vi "Teleop.vi"(0 "Call Context":T10) -> (6 "SubState 3":T4, 8 "SubState 4":T4, 9 "SubState 5":T9, 11 "Loop 3 Data":T5, 13 "Loop 4 Data":T3, 14 "SubState 0":T4=enum."driver control", 15 "Loop 1 Data":T7, 16 "Loop 0 Data":T8, 17 "SubState 1":T4, 18 "Loop 2 Data":T6, 19 "SubState 2":T4)   [LabVIEW 2013]
uses:
  typedefs/subStates.ctl
  <vilib>/Rock Robotics/WPI/DriverStation/WPI_DriverStationDerivedRobotMode.ctl
  typedefs/singleUseSubstate.ctl
  typedefs/Loop Datatypes/Loop 0 Datatype.ctl
  typedefs/Loop Datatypes/Loop 1 Datatype.ctl
  typedefs/Loop Datatypes/Loop 2 Datatype.ctl
  typedefs/Loop Datatypes/Loop 3 Datatype.ctl
  typedefs/Loop Datatypes/Loop 4 Datatype.ctl
  <vilib>/Rock Robotics/WPI/Joystick/WPI_JoystickDevRef.ctl
  <vilib>/Rock Robotics/WPI/Joystick/WPI_JoystickDeviceEnum.ctl
  typedefs/fg_typedef.ctl
  <vilib>/Rock Robotics/WPI/Joystick/WPI_JoystickGetSetRefNum.vi
panel:
  out "Drive to DC":bool
  out "JS2 Button 9":bool
  out "JS3":T1
  out "JS1":T1
  out "JS2":T1
  out "Exit Value":i32=-1
  # "Loop Data and Substates"
  # "Drive Loop"
  # "Unassigned Loop"
  # "Unassigned Loop"
  # "Unassigned Loop"
  # "Unassigned Loop"
  # "Pneumatic Loop"
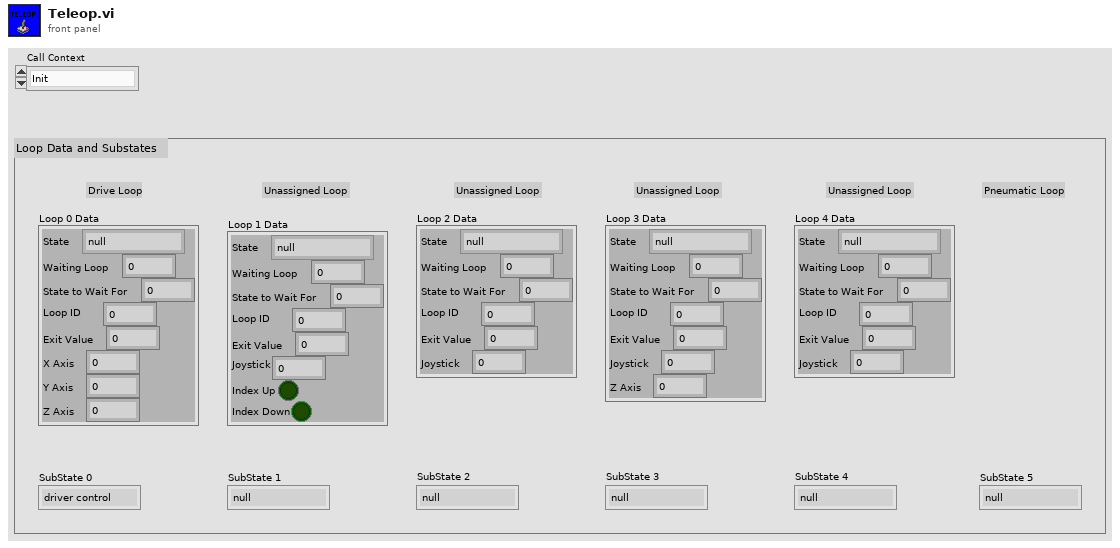
[diagram p1: front panel]
types:
  T1 = typedef "WPI_JoystickDevRef.ctl" = cluster{"Device":T2}
  T2 = typedef "WPI_JoystickDeviceEnum.ctl" = enum16{"USB 1", "USB 2", "USB 3", "USB 4", "Kinect 1", "Kinect 2"}
  T3 = typedef "Loop 4 Datatype.ctl" = cluster{"State":T4, "Waiting Loop":i32, "State to Wait For":i32, "Loop ID":i32, "Exit Value":i32, "Joystick":dbl}
  T4 = typedef "subStates.ctl" = enum16{"null", "wait", "driver control", "auto", "manual override", "hold position", "rotate", "feeder", "shoot", "end"}
  T5 = typedef "Loop 3 Datatype.ctl" = cluster{"State":T4, "Waiting Loop":i32, "State to Wait For":i32, "Loop ID":i32, "Exit Value":i32, "Joystick":dbl, "Z Axis":dbl}
  T6 = typedef "Loop 2 Datatype.ctl" = cluster{"State":T4, "Waiting Loop":i32, "State to Wait For":i32, "Loop ID":i32, "Exit Value":i32, "Joystick":dbl}
  T7 = typedef "Loop 1 Datatype.ctl" = cluster{"State":T4, "Waiting Loop":i32, "State to Wait For":i32, "Loop ID":i32, "Exit Value":i32, "Joystick":dbl, "Index Up":bool, "Index Down":bool}
  T8 = typedef "Loop 0 Datatype.ctl" = cluster{"State":T4, "Waiting Loop":i32, "State to Wait For":i32, "Loop ID":i32, "Exit Value":i32, "X Axis":dbl, "Y Axis":dbl, "Z Axis":dbl}
  T9 = typedef "singleUseSubstate.ctl" = enum16{"null", "wait", "shift high", "shift low"}
  T10 = typedef "WPI_DriverStationDerivedRobotMode.ctl" = enum16{"Init", "Execute", "Stop"}
  T11 = cluster{"axis 1 (x)":dbl, "axis 2 (y)":dbl, "axis 3 (throttle)":dbl, "axis 4":dbl, "axis 5":dbl, "axis 6":dbl}
  T12 = typedef "WPI_JoystickButtonState.ctl" = cluster{"Button 1":bool, "Button 2":bool, "Button 3":bool, "Button 4":bool, "Button 5":bool, "Button 6":bool, "Button 7":bool, "Button 8":bool, "Button 9":bool, "Button 10":bool, "Button 11":bool, "Button 12":bool}
  T13 = typedef "WPI_EncoderDevRef.ctl" = cluster{"DevStatus":errorcluster, "EncoderIndex":T14, "CounterIndex":T15, "DistancePerCount":dbl, "Decoding Type":T16}
  T14 = typedef "FPGA_EncoderIdx.ctl" = enum8{"Enc 0", "Enc 1", "Enc 2", "Enc 3", "Invalid"}
  T15 = typedef "FPGA_CounterCtrSystemIndex.ctl" = enum8{"Ctr 0", "Ctr 1", "Ctr 2", "Ctr 3", "Ctr 4", "Ctr 5", "Ctr 6", "Ctr 7", "Invalid"}
  T16 = typedef "WPI_EncoderType.ctl" = enum16{"1x", "2x", "4x"}
  T17 = typedef "fg_typedef.ctl" = enum16{"Get", "Set"}
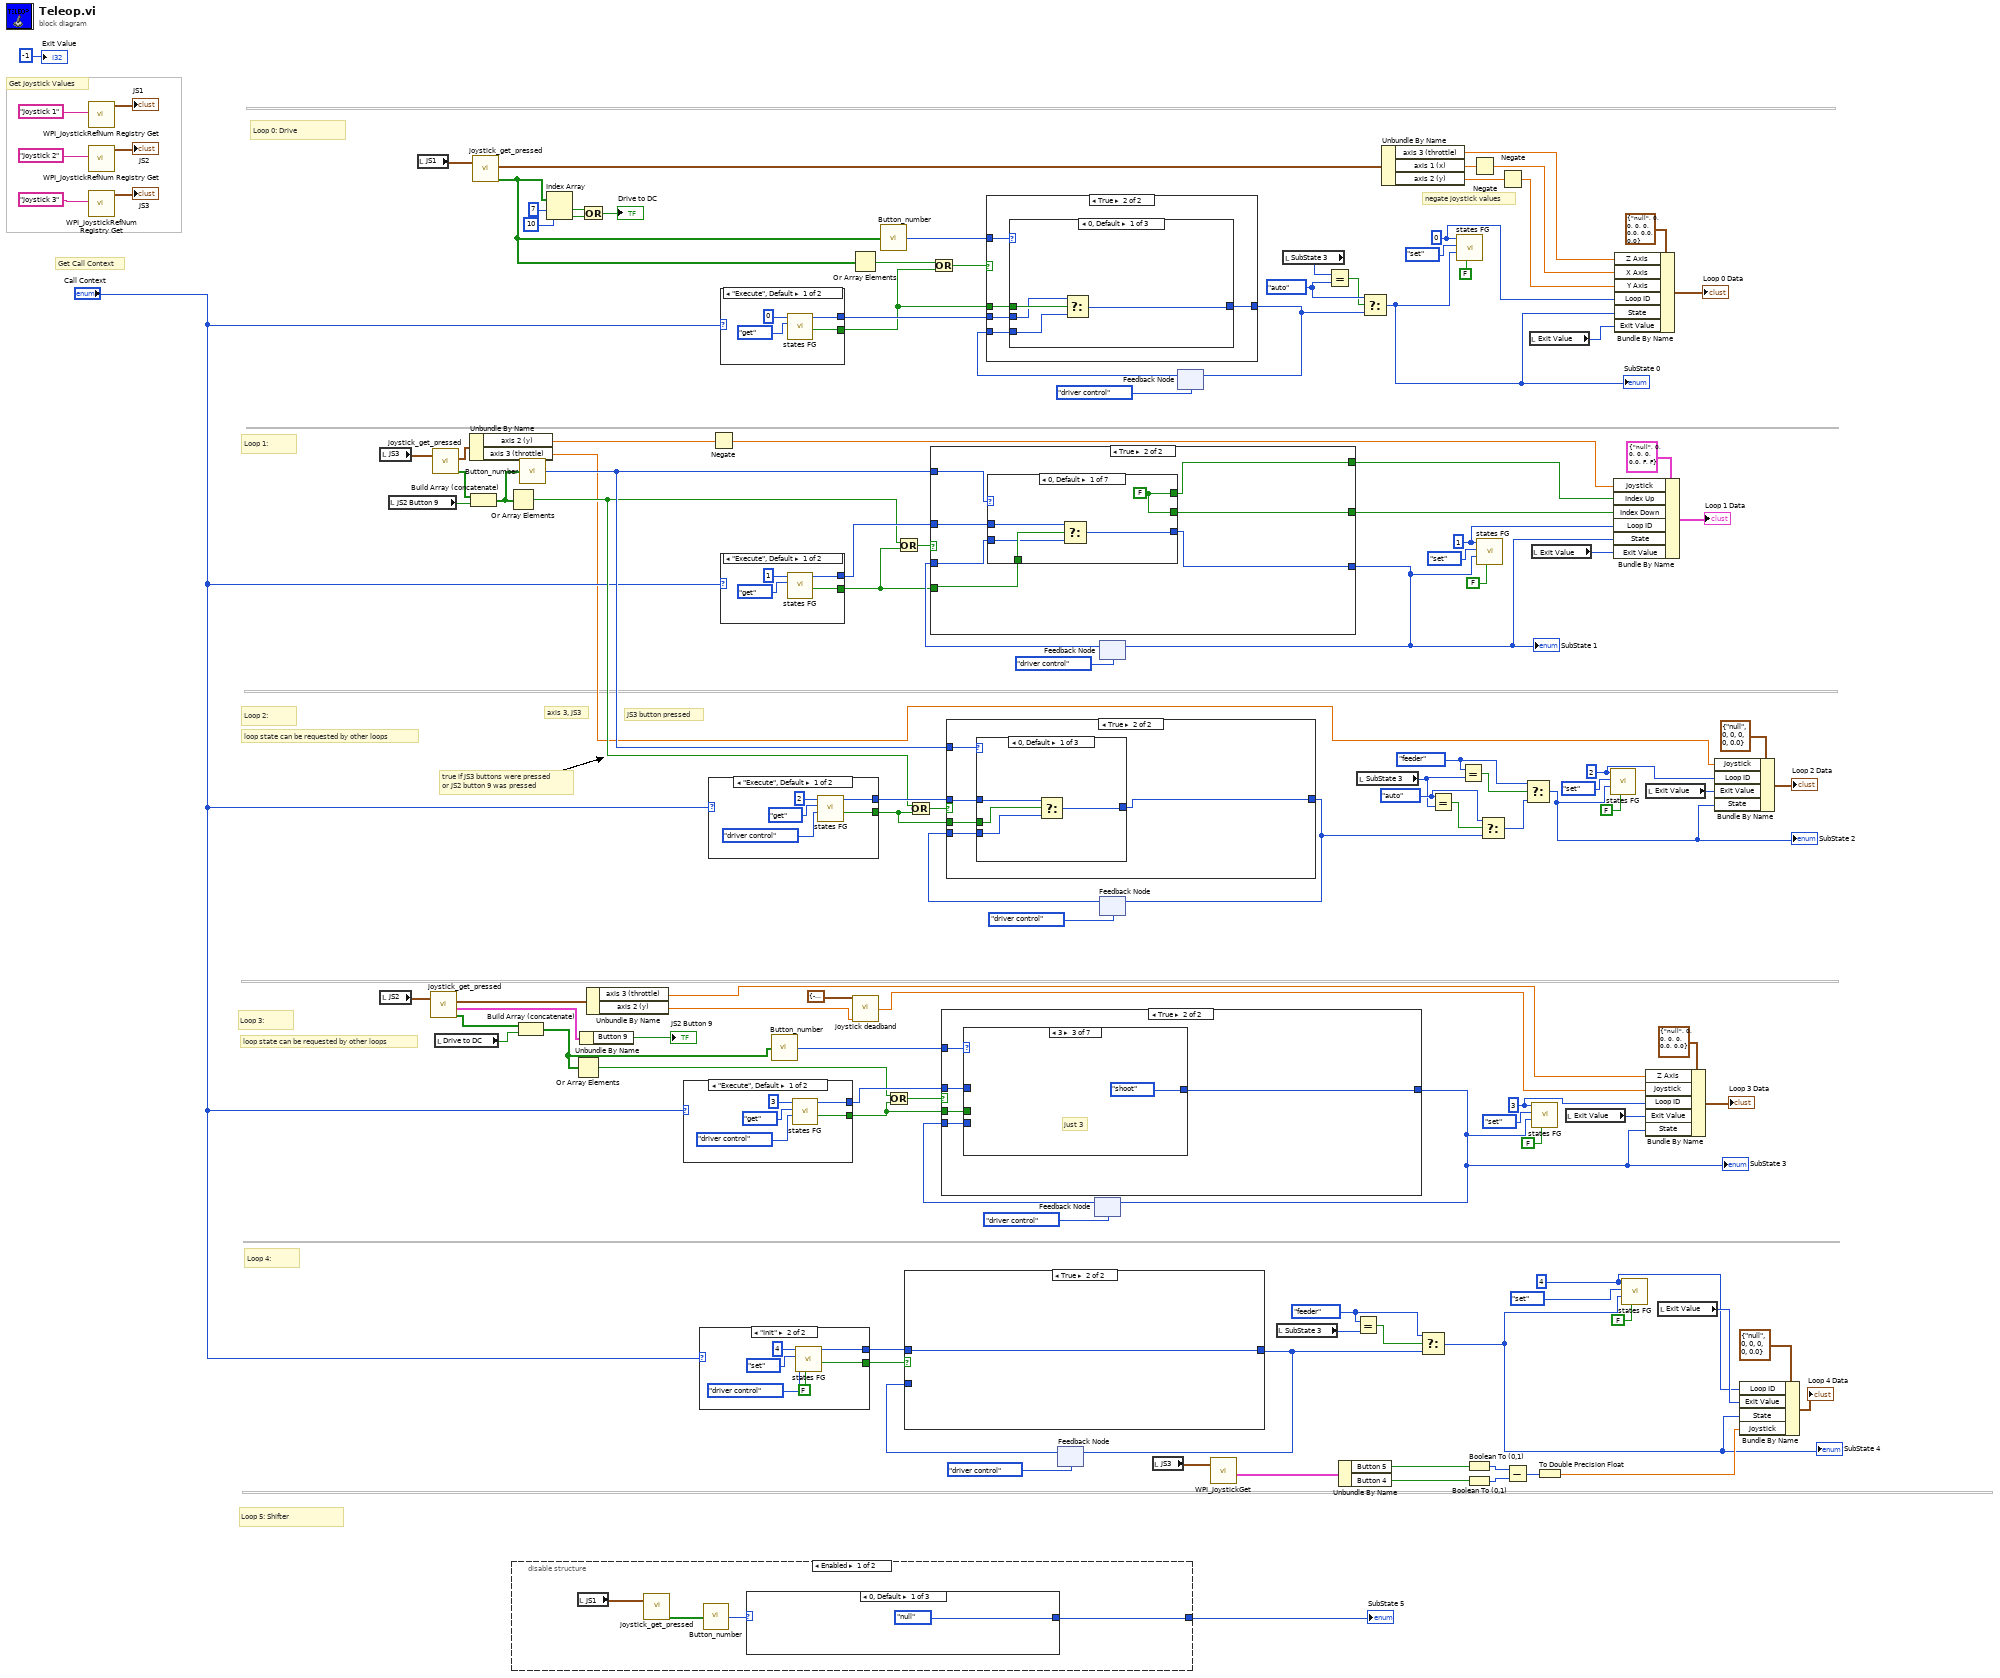
[diagram p0: block diagram]
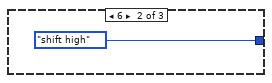
[diagram p2: hidden frame]
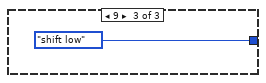
[diagram p3: hidden frame]
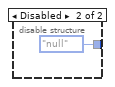
[diagram p4: hidden frame]
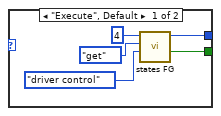
[diagram p6: hidden frame]
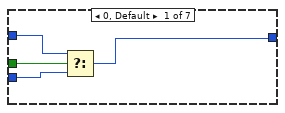
[diagram p8: hidden frame]
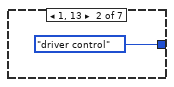
[diagram p9: hidden frame]
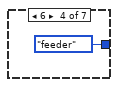
[diagram p10: hidden frame]
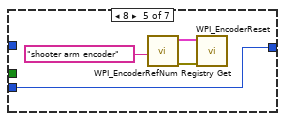
[diagram p11: hidden frame]
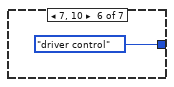
[diagram p12: hidden frame]
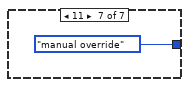
[diagram p13: hidden frame]
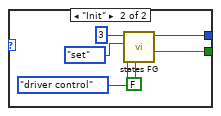
[diagram p14: hidden frame]
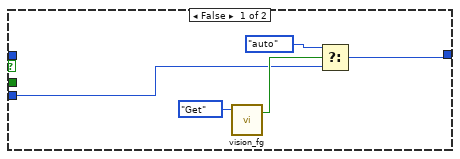
[diagram p15: hidden frame]
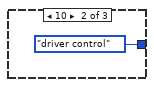
[diagram p16: hidden frame]
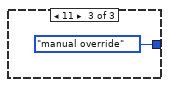
[diagram p17: hidden frame]
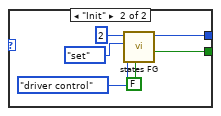
[diagram p18: hidden frame]
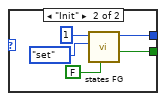
[diagram p19: hidden frame]
diagram:
  w23 = subStates."auto" ("y")
  w26 = subStates."auto" ("x")
  w33 = subStates."feeder" ("x")
  w35 = subStates."feeder" ("x")
  w88 = 4 ("Loop ID")
  w103 = 3 ("Loop ID")
  w104 = 2 ("Loop ID")
  w113 = 1 ("Loop ID")
  w115 = 0 ("Loop ID")
  # "true if JS3 buttons were pressed\nor JS2 button 9 was pressed"
  # "JS3 button pressed"
  # "axis 3, JS3"
  # "negate joystick values"
  # "Get Call Context"
  # "Get Joystick Values"
  # "Loop 4:"
  # "Loop 3:"
  # "loop state can be requested by other loops"
  # "Loop 5: Shifter"
  # "Loop 2:"
  # "Loop 1:"
  # "Loop 0: Drive"
  # "loop state can be requested by other loops"
  n1 = call <vilib>:"WPI_JoystickRefNum Registry Get.vi"("refnum name"="Joystick 1") -> ("JoystickDevRef"=→"JS1":T1)  [unwired: 9 in, 1 out]
  n2 = call <vilib>:"WPI_JoystickRefNum Registry Get.vi"("refnum name"="Joystick 2") -> ("JoystickDevRef"=→"JS2":T1)  [unwired: 9 in, 1 out]
  n3 = call <vilib>:"WPI_JoystickRefNum Registry Get.vi"("refnum name"="Joystick 3") -> ("JoystickDevRef"=→"JS3":T1)  [unwired: 9 in, 1 out]
  n4 = local read "JS3"() -> (w68:T1)
  n5 = local read "JS2"() -> (w46:T1)
  n6 = local read "JS2 Button 9"() -> (w53:bool)
  n7 = local read "JS1"() -> (w69:T1)
  n8 = call "joystick_get_pressed.vi"("JoystickDevRef 2"=w46) -> ("Axes"=w51:T11, "Buttons"=w5:T12, "Buttons Pressed?"=w49:bool[])  [unwired: 1 in, 1 out]
  n9 = call "joystick_get_pressed.vi"("JoystickDevRef 2"=w68) -> ("Axes"=w67:T11, "Buttons Pressed?"=w29:bool[])  [unwired: 1 in, 2 out]
  n10 = local read "Drive to DC"() -> (w8:bool)
  n11 = Unbundle By Name(w67) -> ("axis 2 (y)"=w76:dbl, "axis 3 (throttle)"=w3:dbl)
  n12 = Build Array (concatenate)(w29, w53) -> (w28:bool[])
  n13 = call "joystick_get_pressed.vi"("JoystickDevRef 2"=w69) -> ("Axes"=w75:T11, "Buttons Pressed?"=w14:bool[])  [unwired: 1 in, 2 out]
  n14 = Or Array Elements(Boolean array=w28) -> (logical OR=w56:bool)
  n15 = disable-structure shown="Enabled" {
    disable-tunnel: [w133 singleUseSubstate."null" ("SubState 5")] -> w85
    frame Enabled {
      n16 = local read "JS1"() -> (w132:T1)
      n17 = call "joystick_get_pressed.vi"("JoystickDevRef 2"=w132) -> ("Buttons Pressed?"=w135:bool[])  [unwired: 1 in, 3 out]
      n18 = call "Button_number.vi"("Button Array"=w135) -> ("Button Pressed"=w134:i32)
      n19 = case shown="0, Default" w134 {
        tunnel: [singleUseSubstate."null" ("Enum") singleUseSubstate."shift high" ("Enum") singleUseSubstate."shift low" ("Enum")] -> w133
        frame 0, Default {
        }
        frame 6 {
        }
        frame 9 {
        }
      }
    }
    frame Disabled {
    }
  }
  "SubState 5" <- w85
  n20 = Build Array (concatenate)(w49, w8) -> (w2:bool[])
  n21 = call "Button_number.vi"("Button Array"=w28) -> ("Button Pressed"=w58:i32)
  n22 = Index Array(array=w14, index #1=7 ("index"), index #2=10 ("index")) -> (element #1=w11:bool, element #2=w10:bool)
  n23 = Or Array Elements(Boolean array=w2) -> (logical OR=w50:bool)
  n24 = Unbundle By Name(w5) -> ("Button 9"=→"JS2 Button 9":bool)
  n25 = Or(x=w11, y=w10) -> (x .or. y?=→"Drive to DC":bool)
  n26 = Unbundle By Name(w51) -> ("axis 3 (throttle)"=w16:dbl, "axis 2 (y)"=w19:dbl)
  n27 = case shown="\"Execute\", Default" "Call Context" {
    tunnel: [w142 w148] -> w47
    tunnel: [w140 w145] -> w101
    frame "Execute", Default {
      n28 = call "states FG.vi"("subState in"=subStates."driver control", "menu (get)"=enum16{"set", "get"}."get", "Loop ID"=3) -> ("exit out"=w142:bool, "subState out"=w140:T4)  [unwired: 5 in, 2 out]
    }
    frame "Init" {
      n29 = call "states FG.vi"("exit in"=FALSE, "subState in"=subStates."driver control", "menu (get)"=enum16{"set", "get"}."set", "Loop ID"=3) -> ("exit out"=w148:bool, "subState out"=w145:T4)  [unwired: 4 in, 2 out]
    }
  }
  n30 = case shown="\"Init\"" "Call Context" {
    tunnel: [w153 w159] -> w43
    tunnel: [w151 w156] -> w90
    frame "Execute", Default {
      n31 = call "states FG.vi"("subState in"=subStates."driver control", "menu (get)"=enum16{"set", "get"}."get", "Loop ID"=4) -> ("exit out"=w153:bool, "subState out"=w151:T4)  [unwired: 5 in, 2 out]
    }
    frame "Init" {
      n32 = call "states FG.vi"("exit in"=FALSE, "subState in"=subStates."driver control", "menu (get)"=enum16{"set", "get"}."set", "Loop ID"=4) -> ("exit out"=w159:bool, "subState out"=w156:T4)  [unwired: 4 in, 2 out]
    }
  }
  n33 = case shown="\"Execute\", Default" "Call Context" {
    tunnel: [w164 w170] -> w55
    tunnel: [w162 w167] -> w120
    frame "Execute", Default {
      n34 = call "states FG.vi"("subState in"=subStates."driver control", "menu (get)"=enum16{"set", "get"}."get", "Loop ID"=2) -> ("exit out"=w164:bool, "subState out"=w162:T4)  [unwired: 5 in, 2 out]
    }
    frame "Init" {
      n35 = call "states FG.vi"("exit in"=FALSE, "subState in"=subStates."driver control", "menu (get)"=enum16{"set", "get"}."set", "Loop ID"=2) -> ("exit out"=w170:bool, "subState out"=w167:T4)  [unwired: 4 in, 2 out]
    }
  }
  n36 = Negate(x=w76) -> (-x=w61:dbl)
  n37 = case shown="\"Execute\", Default" "Call Context" {
    tunnel: [w174 w179] -> w65
    tunnel: [w173 w177] -> w118
    frame "Execute", Default {
      n38 = call "states FG.vi"("menu (get)"=enum16{"set", "get"}."get", "Loop ID"=0) -> ("exit out"=w174:bool, "subState out"=w173:T4)  [unwired: 6 in, 2 out]
    }
    frame "Init" {
      n39 = call "states FG.vi"("exit in"=FALSE, "menu (get)"=enum16{"set", "get"}."set", "Loop ID"=0) -> ("exit out"=w179:bool, "subState out"=w177:T4)  [unwired: 5 in, 2 out]
    }
  }
  n40 = case shown="\"Execute\", Default" "Call Context" {
    tunnel: [w183 w188] -> w62
    tunnel: [w182 w186] -> w117
    frame "Execute", Default {
      n41 = call "states FG.vi"("menu (get)"=enum16{"set", "get"}."get", "Loop ID"=1) -> ("exit out"=w183:bool, "subState out"=w182:T4)  [unwired: 6 in, 2 out]
    }
    frame "Init" {
      n42 = call "states FG.vi"("exit in"=FALSE, "menu (get)"=enum16{"set", "get"}."set", "Loop ID"=1) -> ("exit out"=w188:bool, "subState out"=w186:T4)  [unwired: 5 in, 2 out]
    }
  }
  n43 = call "Button_number.vi"("Button Array"=w2) -> ("Button Pressed"=w48:i32)
  n44 = Or Array Elements(Boolean array=w14) -> (logical OR=w66:bool)
  n45 = call "joystick deadband.vi"("Joystick In"=w19, "Deadband Range"=cluster{"Deadband Min":dbl, "Deadband Max":dbl} {"Deadband Min"=-0.05, "Deadband Max"=0.05}) -> ("Joystick Out"=w1:dbl)  [unwired: 4 in]
  n46 = call "Button_number.vi"("Button Array"=w14) -> ("Button Pressed"=w74:i32)
  n47 = Or(x=w50, y=w47) -> (x .or. y?=w52:bool)
  n48 = Or(x=w56, y=w62) -> (x .or. y?=w63:bool)
  n49 = Or(x=w56, y=w55) -> (x .or. y?=w57:bool)
  n50 = Or(x=w66, y=w65) -> (x .or. y?=w64:bool)
  n51 = feedback #1(subStates."driver control" ("Drive SubState")) -> (w93:T4)
  n52 = case shown="True" w43 {
    tunnel: w93 -> [w191 _]
    tunnel: [w191 w192] -> w30
    tunnel: w90 -> [_ w192]
    frame False {
    }
    frame True {
    }
  }
  n53 = feedback-in #1(w30) -> ()
  n54 = feedback #2(subStates."driver control" ("Drive SubState")) -> (w98:T4)
  n55 = case shown="True" w52 {
    tunnel: w98 -> [w193 w194]
    tunnel: [w193 w195] -> w77
    tunnel: w101 -> [_ w196]
    tunnel: w48 -> [_ w198]
    tunnel: w47 -> [_ w197]
    frame False {
    }
    frame True {
      n56 = case shown="3" w198 {
        tunnel: w197 -> [w202 _ _ _ _ _ _]
        tunnel: w194 -> [w201 _ _ _ w206 _ _]
        tunnel: w196 -> [w200 _ _ _ _ _ _]
        tunnel: [w199 subStates."driver control" ("Drive SubState") subStates."shoot" ("Drive SubState") subStates."feeder" ("Drive SubState") w206 subStates."driver control" ("Drive SubState") subStates."manual override" ("Drive SubState")] -> w195
        frame 0, Default {
          n57 = Select(t=w200, s=w202, f=w201) -> (s? t:f=w199:T4)
        }
        frame 1, 13 {
        }
        frame 3 {
          # "just 3"
        }
        frame 6 {
        }
        frame 8 {
          n58 = call <vilib>:"WPI_EncoderRefNum Registry Get.vi"("refnum name"="shooter arm encoder") -> ("error out"=w208:errorcluster, "EncoderDevRef"=w207:T13)  [unwired: 9 in]
          n59 = call <vilib>:"WPI_EncoderReset.vi"("error in (no error)"=w208, "EncoderDevRef"=w207) -> ()  [unwired: 8 in, 2 out]
        }
        frame 7, 10 {
        }
        frame 11 {
        }
      }
    }
  }
  "SubState 3" <- w77
  n60 = feedback-in #2(w77) -> ()
  n61 = feedback #3(subStates."driver control" ("Drive SubState")) -> (w119:T4)
  n62 = case shown="True" w63 {
    tunnel: w119 -> [w212 w218]
    tunnel: [w212 w213] -> w78
    tunnel: w117 -> [_ w219]
    tunnel: w58 -> [_ w217]
    tunnel: w62 -> [_ w216]
    tunnel: [_ w215] -> w60
    tunnel: [_ w214] -> w59
    frame False {
      # "nothing pressed here, move along"
    }
    frame True {
      n63 = case shown="0, Default" w217 {
        tunnel: w219 -> [w223 _ _ _ _ _ _]
        tunnel: w218 -> [w222 _ _ _ _ _ w241]
        tunnel: [w221 subStates."driver control" ("Drive SubState") subStates."driver control" ("Drive SubState") subStates."driver control" ("Drive SubState") subStates."manual override" ("Drive SubState") subStates."driver control" ("Drive SubState") w241] -> w213
        tunnel: w216 -> [w224 _ _ _ _ _ _]
        tunnel: [w220 TRUE FALSE w231 w233 w235 w237] -> w215
        tunnel: [w220 FALSE TRUE w231 w233 w235 w237] -> w214
        frame 0, Default {
          w220 = FALSE
          n64 = Select(t=w223, s=w224, f=w222) -> (s? t:f=w221:T4)
        }
        frame 2 {
        }
        frame 3 {
        }
        frame 6 {
          w231 = FALSE
        }
        frame 9 {
          w233 = FALSE
        }
        frame 8, 10 {
          w235 = FALSE
        }
        frame 13 {
          w237 = FALSE
          n65 = call <vilib>:"WPI_EncoderRefNum Registry Get.vi"("refnum name"="auger encoder") -> ("error out"=w239:errorcluster, "EncoderDevRef"=w238:T13)  [unwired: 9 in]
          n66 = call <vilib>:"WPI_EncoderReset.vi"("error in (no error)"=w239, "EncoderDevRef"=w238) -> ()  [unwired: 8 in, 2 out]
        }
      }
    }
  }
  "SubState 1" <- w78
  n67 = feedback-in #3(w78) -> ()
  n68 = feedback #4(subStates."driver control" ("Drive SubState")) -> (w123:T4)
  n69 = case shown="True" w57 {
    tunnel: w123 -> [w242 w248]
    tunnel: [w243 w247] -> w6
    tunnel: w120 -> [_ w249]
    tunnel: w58 -> [_ w251]
    tunnel: w55 -> [_ w250]
    frame False {
      n70 = call "vision_fg.vi"("Menu"=fg_typedef."Get") -> ("Enabled?"=w245:bool)  [unwired: 2 in, 1 out]
      n71 = Select(t=subStates."auto", s=w245, f=w242) -> (s? t:f=w243:T4)
    }
    frame True {
      n72 = case shown="0, Default" w251 {
        tunnel: w250 -> [w255 _ _]
        tunnel: w249 -> [w254 _ _]
        tunnel: w248 -> [w253 _ _]
        tunnel: [w252 subStates."driver control" ("Drive SubState") subStates."manual override" ("Drive SubState")] -> w247
        frame 0, Default {
          n73 = Select(t=w254, s=w255, f=w253) -> (s? t:f=w252:T4)
        }
        frame 10 {
        }
        frame 11 {
        }
      }
    }
  }
  n74 = feedback-in #4(w6) -> ()
  n75 = local read "JS3"() -> (w45:T1)
  n76 = feedback #5(subStates."driver control" ("Drive SubState")) -> (w125:T4)
  n77 = case shown="True" w64 {
    tunnel: w125 -> [w258 w260]
    tunnel: [w258 w259] -> w17
    tunnel: w118 -> [_ w261]
    tunnel: w74 -> [_ w263]
    tunnel: w65 -> [_ w262]
    frame False {
      # "keep current state, no change necessary"
    }
    frame True {
      n78 = case shown="0, Default" w263 {
        tunnel: w262 -> [w267 _ _]
        tunnel: w261 -> [w266 _ _]
        tunnel: w260 -> [w265 _ w273]
        tunnel: [w264 subStates."driver control" ("Drive SubState") w269] -> w259
        frame 0, Default {
          n79 = Select(t=w266, s=w267, f=w265) -> (s? t:f=w264:T4)
        }
        frame 8, 11 {
          # "put robot drive in driver control"
        }
        frame 7 {
          w270 = subStates."hold position" ("x")
          # "button 7, hold position toggle"
          n80 = Equal?(x=w270, y=w273) -> (x = y?=w272:bool)
          n81 = Select(t=subStates."driver control" ("Drive SubState"), s=w272, f=w270) -> (s? t:f=w269:T4)
        }
      }
    }
  }
  n82 = feedback-in #5(w17) -> ()
  n83 = call <vilib>:"WPI_JoystickGet.vi"("JoystickDevRef"=w45) -> ("Buttons"=w44:T12)  [unwired: 4 in, 2 out]
  n84 = local read "SubState 3"() -> (w32:T4)
  n85 = local read "SubState 3"() -> (w21:T4)
  n86 = Equal?(x=w21, y=w23) -> (x = y?=w22:bool)
  n87 = Unbundle By Name(w44) -> ("Button 5"=w42:bool, "Button 4"=w41:bool)
  n88 = Equal?(x=w33, y=w32) -> (x = y?=w34:bool)
  n89 = local read "SubState 3"() -> (w24:T4)
  n90 = Select(t=w23, s=w22, f=w17) -> (s? t:f=w20:T4)
  "SubState 0" <- w20
  n91 = Unbundle By Name(w75) -> ("axis 3 (throttle)"=w15:dbl, "axis 1 (x)"=w82:dbl, "axis 2 (y)"=w81:dbl)
  n92 = Select(t=w33, s=w34, f=w30) -> (s? t:f=w31:T4)
  "SubState 4" <- w31
  n93 = Equal?(x=w26, y=w24) -> (x = y?=w27:bool)
  n94 = call "states FG.vi"("exit in"=FALSE, "subState in"=w20, "menu (get)"=enum16{"set", "get"}."set", "Loop ID"=w115) -> ()  [unwired: 4 in, 4 out]
  n95 = Equal?(x=w35, y=w24) -> (x = y?=w36:bool)
  n96 = Boolean To (0,1)(Boolean=w42) -> (0, 1=w39:i16)
  n97 = Boolean To (0,1)(Boolean=w41) -> (0, 1=w40:i16)
  n98 = Negate(x=w82) -> (-x=w80:dbl)
  n99 = call "states FG.vi"("exit in"=FALSE, "subState in"=w78, "menu (get)"=enum16{"set", "get"}."set", "Loop ID"=w113) -> ()  [unwired: 4 in, 4 out]
  n100 = Select(t=w26, s=w27, f=w6) -> (s? t:f=w25:T4)
  n101 = Negate(x=w81) -> (-x=w79:dbl)
  n102 = Subtract(x=w39, y=w40) -> (x-y=w38:i16)
  n103 = Select(t=w35, s=w36, f=w25) -> (s? t:f=w7:T4)
  "SubState 2" <- w7
  n104 = local read "Exit Value"() -> (w111:i32)
  n105 = local read "Exit Value"() -> (w110:i32)
  n106 = call "states FG.vi"("exit in"=FALSE, "subState in"=w77, "menu (get)"=enum16{"set", "get"}."set", "Loop ID"=w103) -> ()  [unwired: 4 in, 4 out]
  n107 = To Double Precision Float(number=w38) -> (double precision float=w37:dbl)
  n108 = local read "Exit Value"() -> (w102:i32)
  n109 = call "states FG.vi"("exit in"=FALSE, "subState in"=w7, "menu (get)"=enum16{"set", "get"}."set", "Loop ID"=w104) -> ()  [unwired: 4 in, 4 out]
  n110 = Bundle By Name(cluster=T7 {"State"=enum."null", "Waiting Loop"=0, "State to Wait For"=0, "Loop ID"=0, "Exit Value"=0, "Joystick"=0.0, "Index Up"=FALSE, "Index Down"=FALSE} ("Cluster"), "Joystick"=w61, "Index Up"=w60, "Index Down"=w59, "Loop ID"=w113, "State"=w78, "Exit Value"=w110) -> (→"Loop 1 Data":T7)
  n111 = Bundle By Name(cluster=T8 {"State"=enum."null", "Waiting Loop"=0, "State to Wait For"=0, "Loop ID"=0, "Exit Value"=0, "X Axis"=0.0, "Y Axis"=0.0, "Z Axis"=0.0} ("Cluster"), "Z Axis"=w15, "X Axis"=w80, "Y Axis"=w79, "Loop ID"=w115, "State"=w20, "Exit Value"=w111) -> (→"Loop 0 Data":T8)
  n112 = call "states FG.vi"("exit in"=FALSE, "subState in"=w31, "menu (get)"=enum16{"set", "get"}."set", "Loop ID"=w88) -> ()  [unwired: 4 in, 4 out]
  n113 = Bundle By Name(cluster=T5 {"State"=enum."null", "Waiting Loop"=0, "State to Wait For"=0, "Loop ID"=0, "Exit Value"=0, "Joystick"=0.0, "Z Axis"=0.0} ("Loop 3 Data"), "Z Axis"=w16, "Joystick"=w1, "Loop ID"=w103, "Exit Value"=w102, "State"=w77) -> (→"Loop 3 Data":T5)
  n114 = local read "Exit Value"() -> (w105:i32)
  n115 = local read "Exit Value"() -> (w89:i32)
  n116 = Bundle By Name(cluster=T6 {"State"=enum."null", "Waiting Loop"=0, "State to Wait For"=0, "Loop ID"=0, "Exit Value"=0, "Joystick"=0.0} ("Loop 2 Data"), "Joystick"=w3, "Loop ID"=w104, "Exit Value"=w105, "State"=w7) -> (→"Loop 2 Data":T6)
  n117 = Bundle By Name(cluster=T3 {"State"=enum."null", "Waiting Loop"=0, "State to Wait For"=0, "Loop ID"=0, "Exit Value"=0, "Joystick"=0.0} ("Loop 4 Data"), "Loop ID"=w88, "Exit Value"=w89, "State"=w31, "Joystick"=w37) -> (→"Loop 4 Data":T3)
  "Exit Value" <- -1 ("Exit Value")
